vi "Pre Loop Init.vi"(8 "error in (no error)":errorcluster, 11 "Ref In":refnum<vi>) -> (0 "error out":errorcluster, 3 "Event Registration Refnum":refnum<event-registration>)   [LabVIEW 2020, in "UI.lvlib"]
uses:
  UI.lvlib
  Private Controls/Element.ctl
  Private Controls/Module Action.ctl
  Queue FGV Action.ctl
  Architecture Support/Architecture Support.lvlib
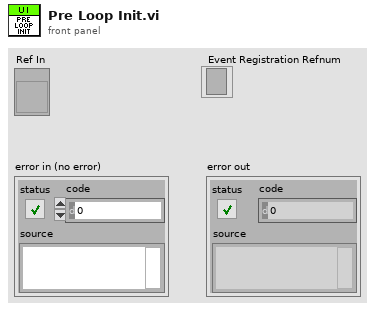
[diagram p1: front panel]
types:
  T1 = typedef "UI.lvlib/Queue FGV Action.ctl" = enum16{"Get", "Set", "Release"}
  T2 = typedef "UI.lvlib/Element.ctl" = cluster{"Action":T3, "Data":variant}
  T3 = typedef "UI.lvlib/Module Action.ctl" = enum16{"Initialise Module", "Connect", "Setup", "Pause", "Start", "Search", "Set IP", "Count Call", "Update Progress Bar", "Update UI", "Stop", "Post Results", "Wait: Time Elapsed", "Error", "Exit"}
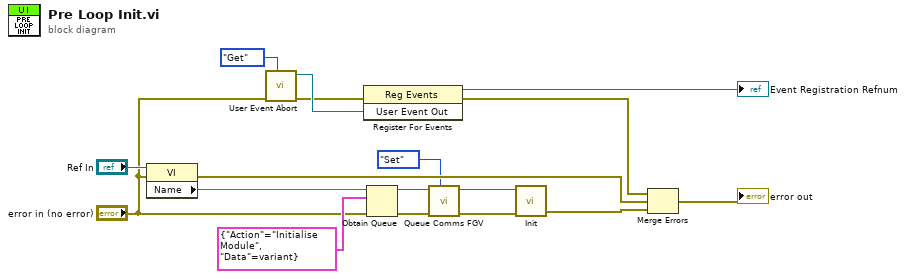
[diagram p0: block diagram]
diagram:
  n1 = property class="VI"(reference="Ref In", error in="error in (no error)") -> (error out=w3:errorcluster, "Name"=w10:string)  [unwired: 1 out]
  n2 = call "User Event Abort.vi"("Enum"=enum16{"Create", "Destroy", "Get"}."Get", "error in (no error)"="error in (no error)") -> ("error out"=w16:errorcluster, "User Event Out"=w17:refnum<user-event>)  [unwired: 8 in]
  n3 = register-events(error in=w16, w17) -> (reference out=→"Event Registration Refnum":refnum<event-registration>, error out=w14:errorcluster)  [unwired: 1 in]
  n4 = Obtain Queue(name (unnamed)=w10, element data type=T2 {"Action"=enum."Initialise Module", "Data"=variant} ("Element"), error in (no error)="error in (no error)") -> (queue out=w11:refnum<queue>, error out=w9:errorcluster)  [unwired: 2 in, 1 out]
  n5 = call "Queue Comms FGV.vi"("Action"=Queue_FGV_Action."Set", "error in (no error)"=w9, "queue In"=w11) -> ("error out"=w7:errorcluster, "queue In"=w6:refnum<queue>)  [unwired: 7 in]
  n6 = call "Init.vi"("error in (no error)"=w7, "Data"=w6) -> ("error out"=w2:errorcluster)  [unwired: 9 in]
  n7 = Merge Errors(w14, w3, w2) -> (→"error out":errorcluster)
